vi "LecturaMordasses.vi"(10 "Clau":string, 11 "NMordasses":u8) -> (2 "Mordasses":T1(array[cluster]) {"ID_M" items=["Nº1", "Nº2", "Nº4", "Nº8", "Nº9", "Nº11", "Nº12", "Nº 14", "CUERNO_CAZA", "P 210-210", "PLATO 200", "DEF_USER_1", "DEF_USER_2", "DEF_USER_3", "DEF_USER_4", "NO_PRESENTE"]})   [LabVIEW 2017]
uses:
  <vilib>/registry/registry.llb/Registry RtKey.ctl
  <vilib>/registry/registry.llb/Read Registry Value Simple STR.vi
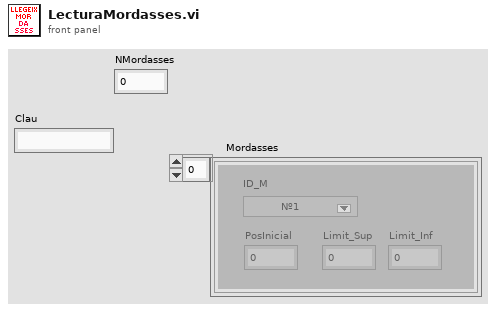
[diagram p1: front panel]
types:
  T1 = cluster{"ID_M":u16, "PosInicial":dbl, "Limit_Sup":dbl, "Limit_Inf":dbl}[]
  T2 = typedef "Registry RtKey.ctl" = enum32{"HKEY_CLASSES_ROOT", "HKEY_CURRENT_USER", "HKEY_LOCAL_MACHINE", "HKEY_USERS", "HKEY_PERFORMANCE_DATA", "HKEY_CURRENT_CONFIG", "HKEY_DYN_DATA"}
  T3 = cluster{"ID_M":u16, "PosInicial":dbl, "Limit_Sup":dbl, "Limit_Inf":dbl}
  T4 = typedef "Registry refnum.ctl" = refnum<k1>
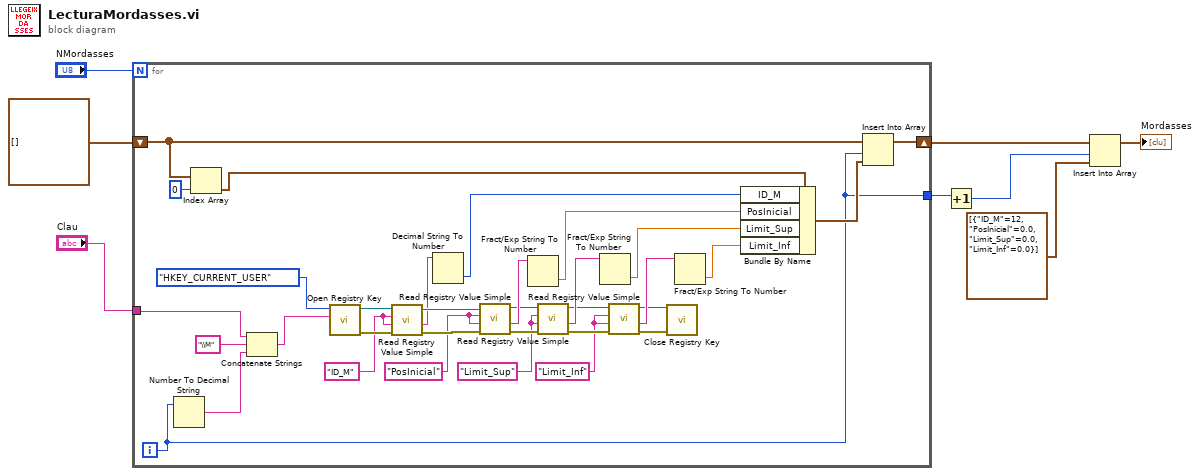
[diagram p0: block diagram]
diagram:
  n1 = for {
    N: "NMordasses" -> [_]
    tunnel: "Clau" -> [w40]
    shift-right: [w34] -> w5
    shift-left: T1 [] ("Mordasses") -> [w30]
    tunnel: [w9] -> w2
    i -> [w9]
    w15 = "Limit_Inf" ("value")
    w20 = "Limit_Sup" ("value")
    w25 = "PosInicial" ("value")
    w33 = "ID_M" ("value")
    n2 = Number To Decimal String(number=w9) -> (decimal integer string=w37:string)  [unwired: 1 in]
    n3 = Index Array(array=w30, index=0) -> (element=w28:T3)
    n4 = Concatenate Strings(w40, "\\M" ("string"), w37) -> (w39:string)
    n5 = call <vilib>:"Open Registry Key.vi"("subkey"=w39, "root key (HKEY_LOCAL_MACHINE)"=Registry_RtKey."HKEY_CURRENT_USER") -> ("error out"=w35:errorcluster, "refnum out"=w36:T4)  [unwired: 8 in]
    n6 = call-poly <vilib>:"Read Registry Value Simple.vi"("error in (no error)"=w35, "default data"=w33, "value"=w33, "refnum"=w36) -> ("error out"=w26:errorcluster, "String/Binary data"=w31:string, "refnum out"=w32:T4)  [unwired: 2 in, 1 out]
    n7 = Decimal String To Number(string=w31) -> (number=w27:i32)  [unwired: 2 in, 1 out]
    n8 = call-poly <vilib>:"Read Registry Value Simple.vi"("error in (no error)"=w26, "default data"=w25, "value"=w25, "refnum"=w32) -> ("error out"=w22:errorcluster, "String/Binary data"=w24:string, "refnum out"=w21:T4)  [unwired: 2 in, 1 out]
    n9 = Fract/Exp String To Number(string=w24) -> (number=w23:dbl)  [unwired: 3 in, 1 out]
    n10 = call-poly <vilib>:"Read Registry Value Simple.vi"("error in (no error)"=w22, "default data"=w20, "value"=w20, "refnum"=w21) -> ("error out"=w16:errorcluster, "String/Binary data"=w19:string, "refnum out"=w17:T4)  [unwired: 2 in, 1 out]
    n11 = Fract/Exp String To Number(string=w19) -> (number=w18:dbl)  [unwired: 3 in, 1 out]
    n12 = call-poly <vilib>:"Read Registry Value Simple.vi"("error in (no error)"=w16, "default data"=w15, "value"=w15, "refnum"=w17) -> ("error out"=w10:errorcluster, "String/Binary data"=w14:string, "refnum out"=w11:T4)  [unwired: 2 in, 1 out]
    n13 = call <vilib>:"Close Registry Key.vi"("error in (no error)"=w10, "refnum"=w11) -> ()  [unwired: 5 in, 1 out]
    n14 = Fract/Exp String To Number(string=w14) -> (number=w13:dbl)  [unwired: 3 in, 1 out]
    n15 = Bundle By Name(cluster=w28, "ID_M"=w27, "PosInicial"=w23, "Limit_Sup"=w18, "Limit_Inf"=w13) -> (w12:T3)
    n16 = Insert Into Array(array=w30, index=w9, new element=w12) -> (w34:T1)
  }
  n17 = Increment(x=w2) -> (x+1=w1:i32)
  n18 = Insert Into Array(array=w5, index=w1, new element=T1 [{"ID_M"=12, "PosInicial"=0.0, "Limit_Sup"=0.0, "Limit_Inf"=0.0}] ("Mordasses")) -> (→"Mordasses":T1)
